vi "add Cyclone Image.vi"(7 "aFile":string, 8 "error in":errorcluster, 9 "replaceImageOfSameDescription":bool, 10 "selectedMediaType":u32, 11 "cycloneHandle":u32) -> (0 "error out":errorcluster, 3 "function return":u32, 5 "aFile out":string)   [LabVIEW 2021, in "CycloneControlSDK.lvlib"]
doc: "extern \"C\" uint32_t _cdecl addCycloneImage(uint32_t cycloneHandle, uint32_t selectedMediaType, bool replaceImageOfSameDescription, char *aFile);"
uses:
  CycloneControlSDK.lvlib
  CycloneControlSDK_64.dll
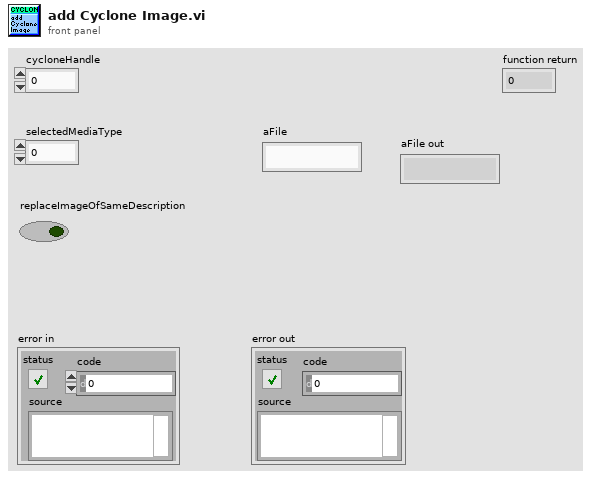
[diagram p1: front panel]
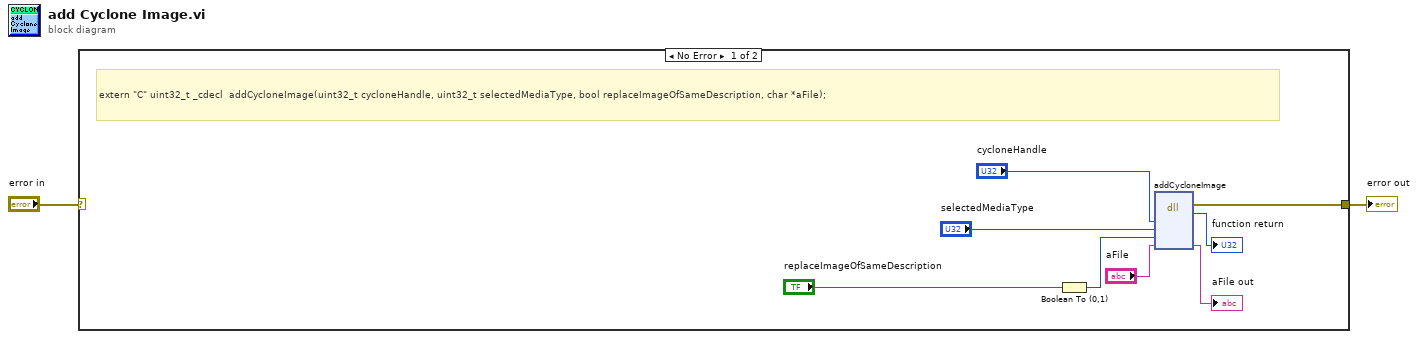
[diagram p0: block diagram]
diagram:
  n1 = case shown="No Error" "error in" {
    selector: "error in" -> [_ w11]
    tunnel: [w3 w11] -> w1
    frame No Error {
      # "extern \"C\" uint32_t _cdecl  addCycloneImage(uint32_t cycloneHandle, uint32_t selectedMediaType, bool replaceImageOfSameDescription, char *aFile);"
      n2 = Boolean To (0,1)(Boolean="replaceImageOfSameDescription") -> (0, 1=w7:i16)
      n3 = dll-call lib="C:/PEMicro/cyclone/cycloneControl/controlsdk/examples/labview2018/user.lib/CycloneControlSDK/CycloneControlSDK_64.dll" fn="addCycloneImage"("cycloneHandle"="cycloneHandle", "selectedMediaType"="selectedMediaType", "replaceImageOfSameDescription"=w7, "aFile"="aFile") -> (error out=w3:errorcluster, "return type"=→"function return":u32, "aFile"=→"aFile out":string)  [unwired: 6 in, 1 out]
    }
    frame Error {
    }
  }
  "error out" <- w1
